vi "M.SWizRot.vi"(8 "error in (no error)":errorcluster, 11 "Microscope in":refnum<class "Microscope.lvclass">) -> (0 "error out":errorcluster, 3 "Microscope out":refnum<class "Microscope.lvclass">)   [LabVIEW 2012, in "Microscope.lvclass"]
uses:
  classes/Microscope.lvclass
  typedefs/Scan Type.ctl
  typedefs/DetectorType.ctl
  typedefs/Move Type.ctl
  classes/Microscope.lvclass/Microscope.ctl
  Spectrometer/SpectrometerSpectraWiz.llb/StellarNet Globals.vi
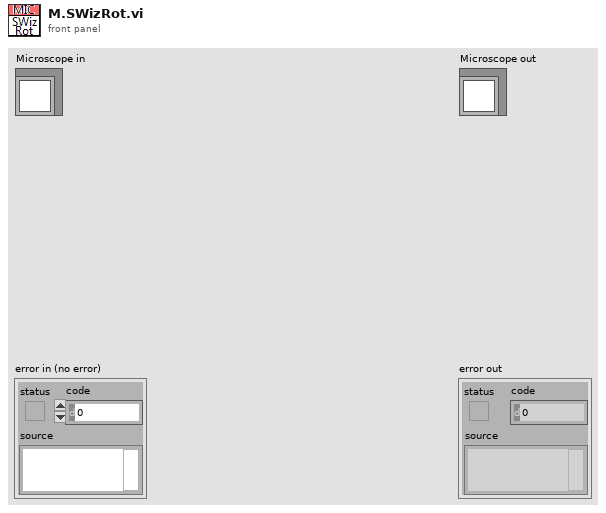
[diagram p1: front panel]
types:
  T1 = typedef "Move Type.ctl" = enum16{"None", "Continuous", "Discrete"}
  T2 = typedef "DetectorType.ctl" = enum16{"PMT", "SpectraWiz"}
  T3 = typedef "Scan Type.ctl" = enum16{"None", "Point", "Full Image Continuous", "Full Image Grab"}
  T4 = typedef "ScanMode.ctl" = enum16{"None", "Continuous", "Point Scan (CH3 cursor)", "Point Scan Move (CH3 cursor)", "Grab", "Grab Move Stage", "Grab Move Z-stage", "Cont. Move Z-stage", "Spec Move Stage", "Spec Move Cont", "Surf Calib"}
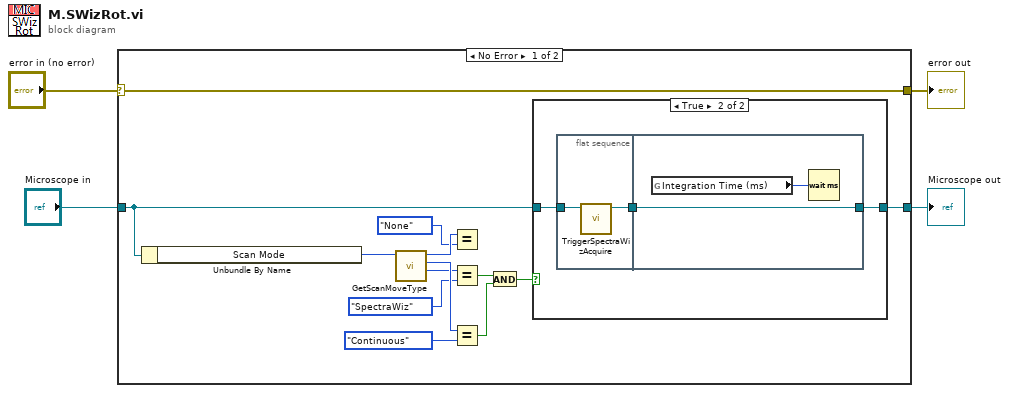
[diagram p0: block diagram]
diagram:
  n1 = case shown="No Error" "error in (no error)" {
    selector: "error in (no error)" -> [w17 w27]
    tunnel: [w17 w27] -> w3
    tunnel: [w5 w26] -> w1
    tunnel: "Microscope in" -> [w6 w26]
    frame No Error {
      n2 = Unbundle By Name(w6) -> ("Scan Mode"=w16:T4)
      n3 = call "GetScanMoveType.vi"("Scan Mode"=w16) -> ("Detector"=w14:T2, "Move Type"=w15:T1, "Scan Type"=w13:T3)  [unwired: 8 in]
      n4 = Equal?(x=w13, y=Scan_Type."None") -> ()  [unwired: 1 out]
      n5 = Equal?(x=w14, y=DetectorType."SpectraWiz") -> (x = y?=w9:bool)
      n6 = Equal?(x=w15, y=Move_Type."Continuous") -> (x = y?=w8:bool)
      n7 = And(x=w9, y=w8) -> (x .and. y?=w7:bool)
      n8 = case shown="True" w7 {
        tunnel: w6 -> [w18 w21]
        tunnel: [w18 w20] -> w5
        frame False {
        }
        frame True {
          n9 = flat-sequence {
            tunnel: w21 -> [w23]
            tunnel: [w22] -> w19
            tunnel: [w25] -> w20
            tunnel: w19 -> [w25]
            frame #0 {
              n10 = call "TriggerSpectraWizAcquire.vi"("Microscope in"=w23) -> ("Microscope out"=w22:refnum<class "Microscope.lvclass">)  [unwired: 9 in, 1 out]
            }
            frame #1 {
              n11 = global read "StellarNet Globals.vi" "Integration Time (ms)"() -> (w24:i32)
              n12 = Wait (ms)(milliseconds to wait=w24) -> ()  [unwired: 1 out]
            }
          }
        }
      }
    }
    frame Error {
    }
  }
  "error out" <- w3
  "Microscope out" <- w1
